vi "OEE_SCREEN_2_map_worst_ok_count_to_cluster.vi"(11 "worst_ok_record":string[](array[string])) -> (2 "performance":string, 3 "station":string)   [LabVIEW 2019]
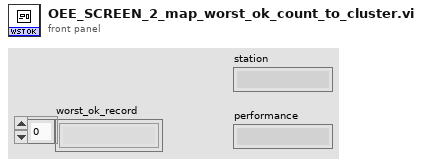
[diagram p1: front panel]
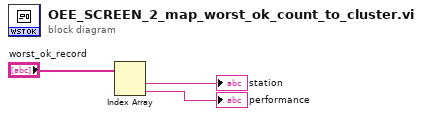
[diagram p0: block diagram]
diagram:
  n1 = Index Array(array="worst_ok_record") -> (element #1=→"station":string, element #2=→"performance":string)  [unwired: 2 in]
